vi "airyscan.vi"() -> ()   [LabVIEW 2015]
uses:
  <vilib>/vision/Image Controls.llb/IMAQ Image.ctl
  Control cluster 1.ctl
  Control digital.ctl
  camera.ctl
  <vilib>/vision/NI_Vision_Development_Module.lvlib
panel:
  out "error in (no error) 3":errorcluster
  out "Frame Index":i32
  in  "piezol":T1
  out "output cluster":T2
  in  "stop":bool
  out "picture frame count":i32
  out "one frame#":dbl
  out "image array":T3[](array[typedef])
  out "Image 4":T3(plugin-control)
  out "Slide":u8(slide) scale=0.0..21.0
  out "y width":dbl
  out "x width":dbl
  out "flyback flag":bool=TRUE
  out "actual number of samples written per channel":u32
  out "flyback step":dbl
  out "actual exposure time":dbl
  out "selected path":path
  out "frame #":u16
  out "y#":dbl
  out "x#":dbl
  out "buffer page size":i32
  in  "save":bool
  out "Signal":u32[](array[numeric])
  in  "digital galvo":T4={" galvo offset"=32427.26, "flyback step"=20.0} {"flyback step" min=0.0 max=10.0 step=0.1; "galvo offset" min=0.0 max=10.0 step=0.1}
  in  "p Cluster":T5={"exposure time"=3.8e-05, "frame #"=2, "x#"=512.0, "y#"=512.0, "x step size"=0.0, "y step size"=0.0, "buffer page size"=1000.0} {"buffer page size" min=0.0 max=2044.0 step=4.0; "y step size" format="%.6f"; "x step size" format="%.6f"; "frame #" min=1 max=2048 step=1; "exposure time" min=0.0 max=10.0 step=0.1}
  out "camera handle":u32
  out "buffer array":T3[](array[typedef])
  in  "error in (no error) 2":errorcluster {"code" format="%.0x"}
  out "Camera Details":T6
  in  "abort":bool
  in  "start":bool
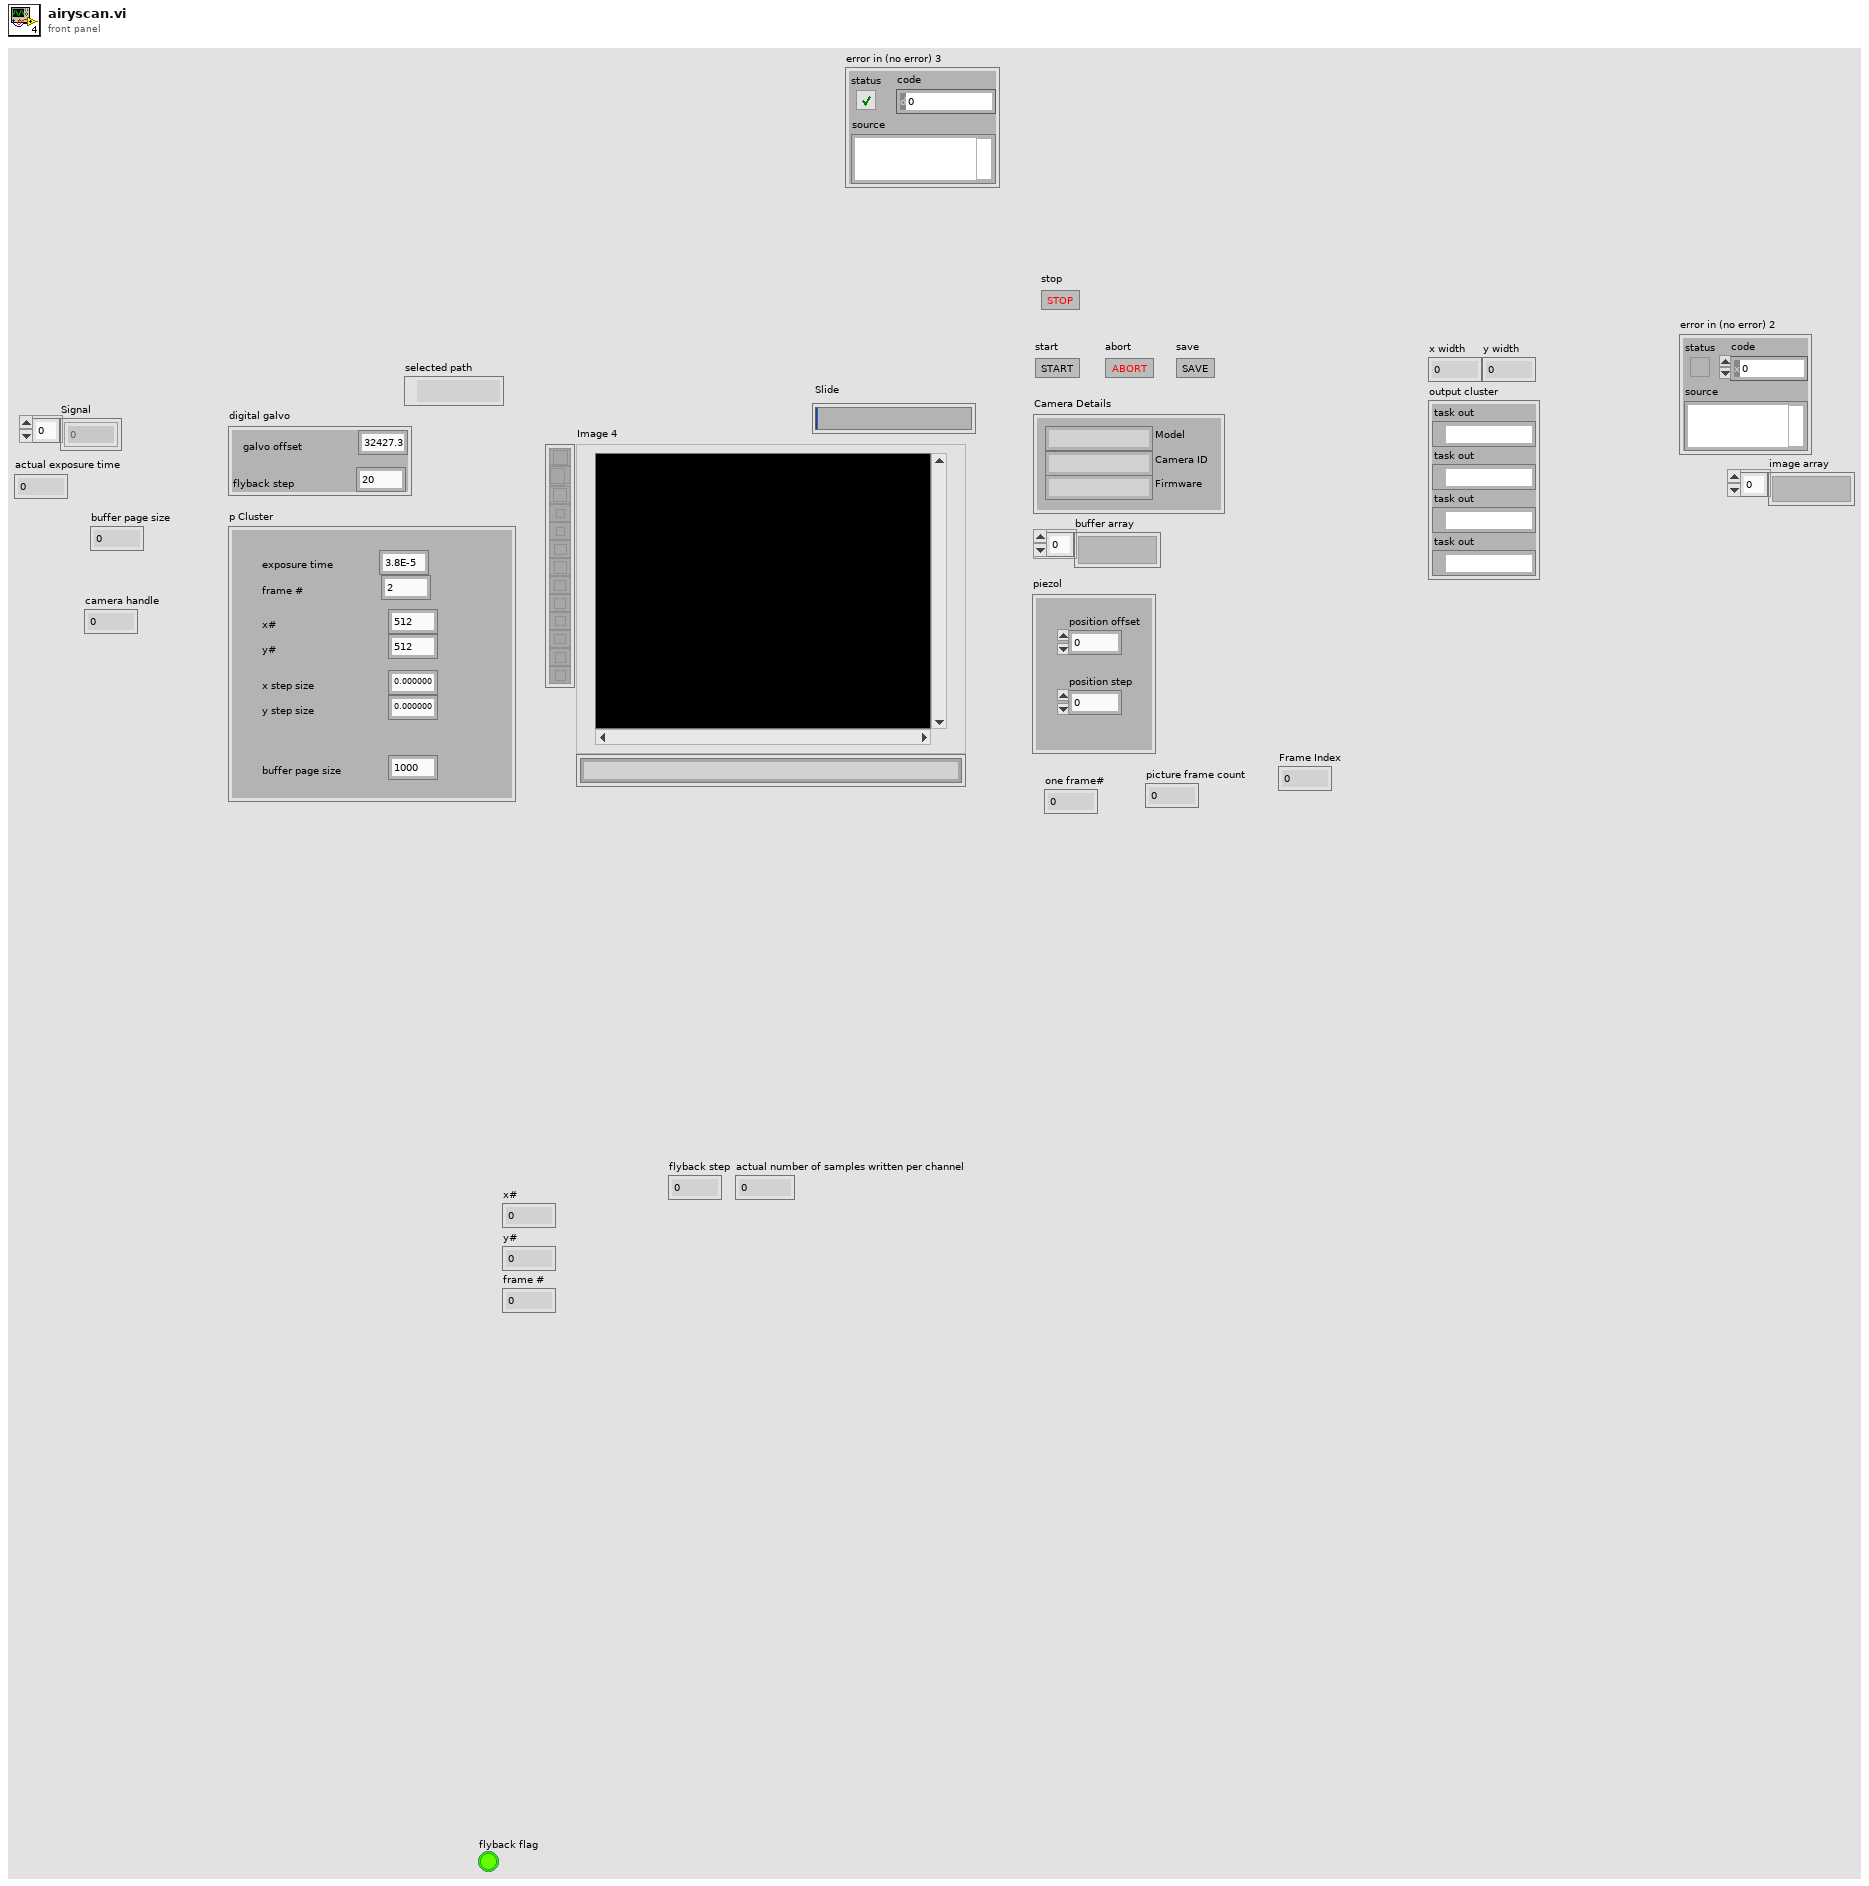
[diagram p1: front panel]
types:
  T1 = cluster{"position offset":dbl, "position step":dbl}
  T2 = cluster{"task out":refnum<k21>, "task out":refnum<k21>, "task out":refnum<k21>, "task out":refnum<k21>}
  T3 = typedef "IMAQ Image.ctl" = refnum<image>
  T4 = typedef "Control digital.ctl" = cluster{" galvo offset":dbl, "flyback step":dbl}
  T5 = typedef "Control cluster 1.ctl" = cluster{"exposure time":dbl, "frame #":u16, "x#":dbl, "y#":dbl, "x step size":dbl, "y step size":dbl, "buffer page size":dbl}
  T6 = cluster{"Model":string, "Camera ID":string, "Firmware":string}
  T7 = typedef "camera.ctl" = enum16{"stop", "state0-initialize", "calculate waveform", "wait for action", "state1-set", "state2-capture", "exit"}
  T8 = cluster{"Rows Per Strip":i32, "Photometric":i32, "Compression Type":i32}
  T9 = typedef "Image Type" = u32
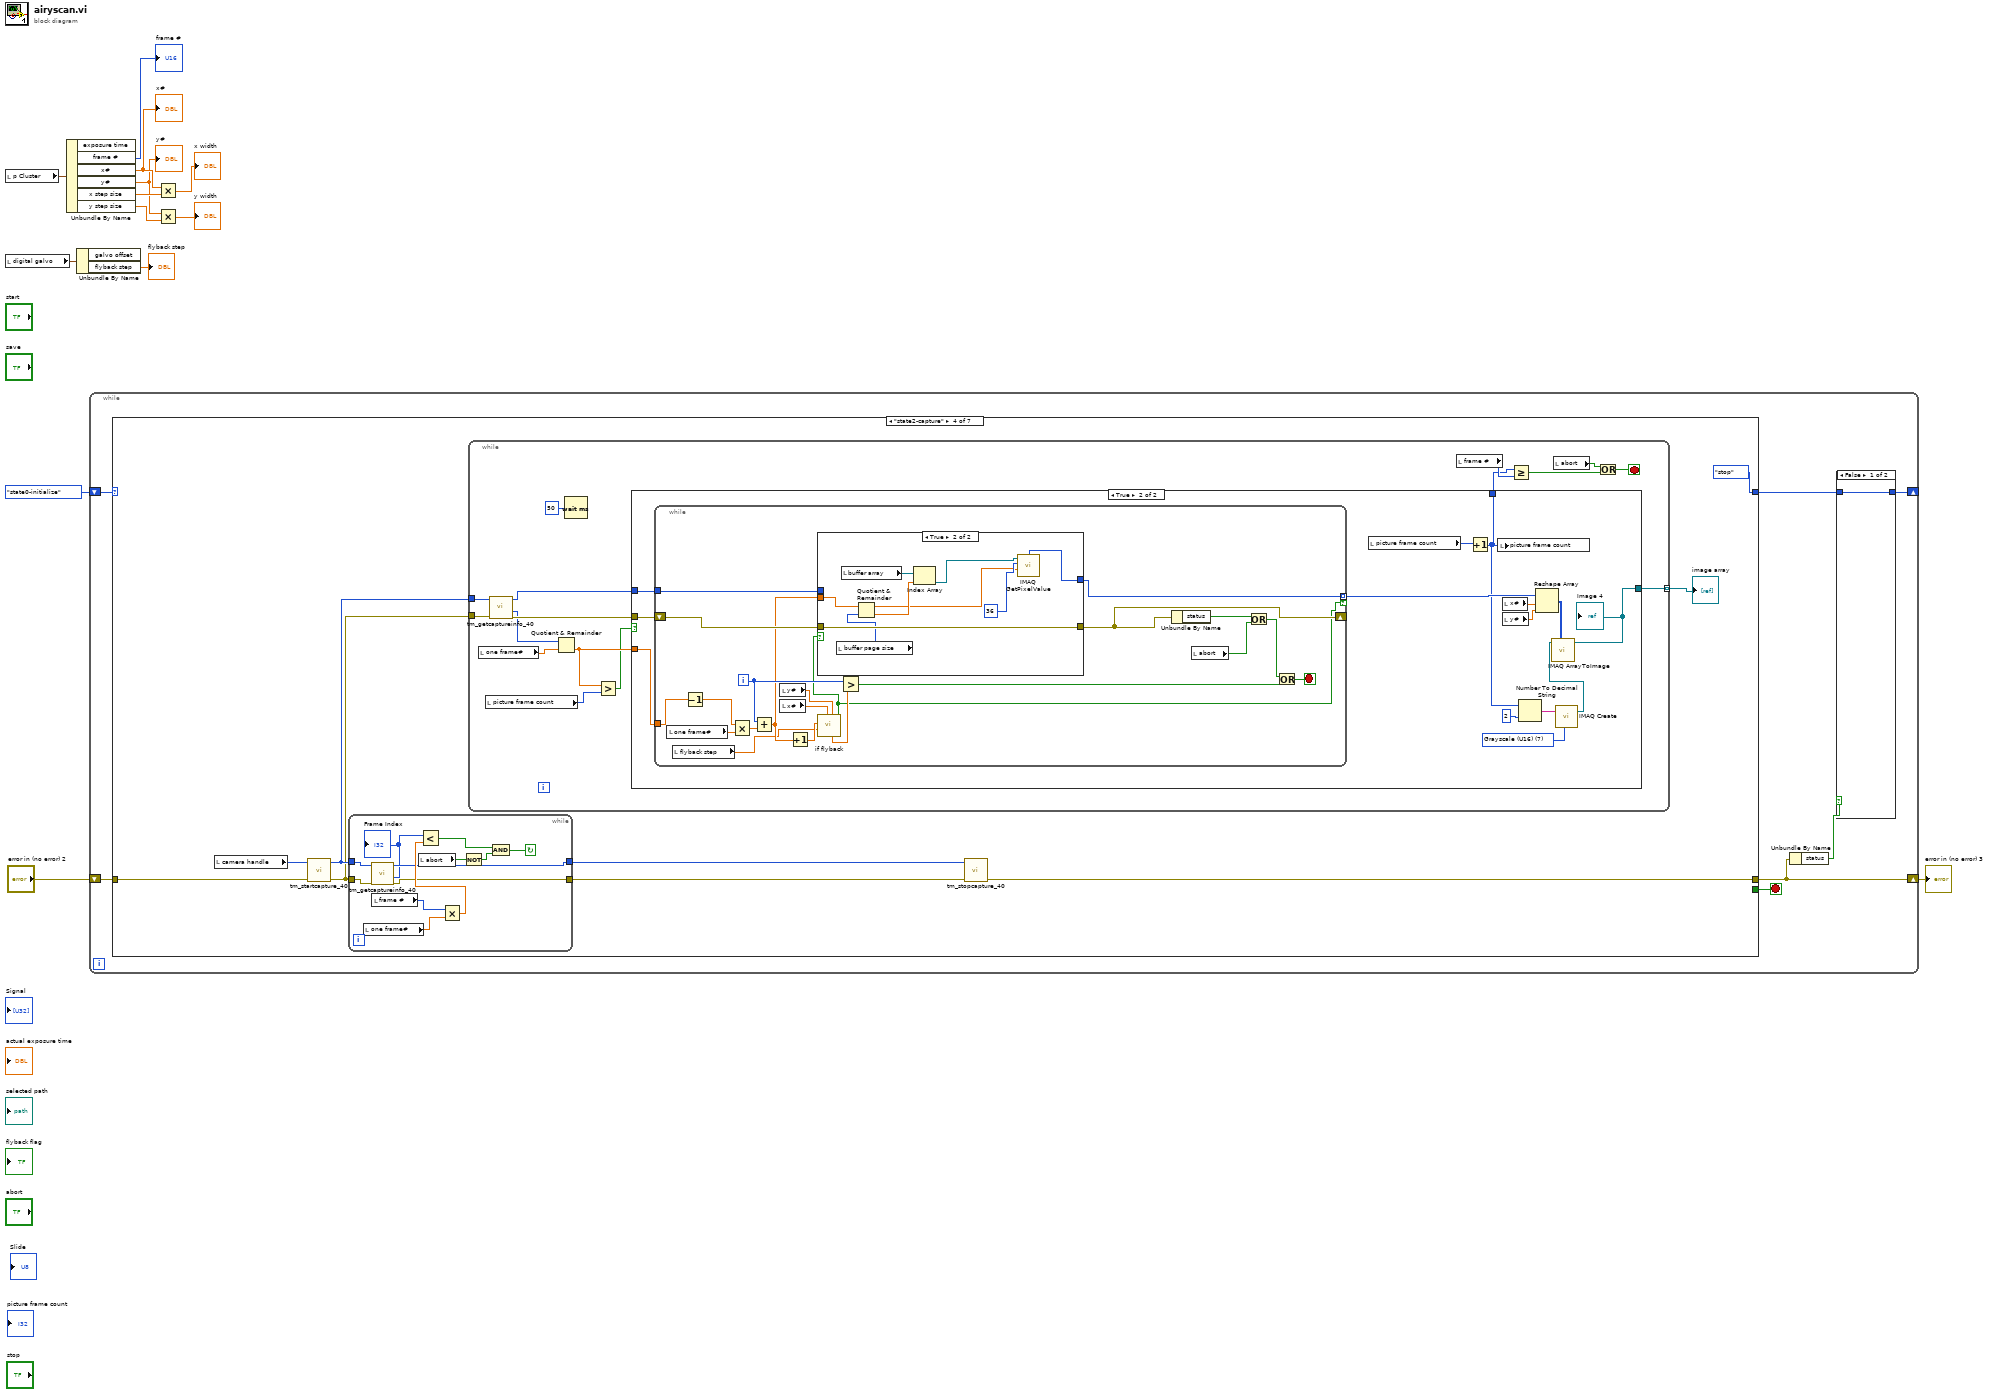
[diagram p0: block diagram]
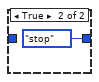
[diagram p2: hidden frame]
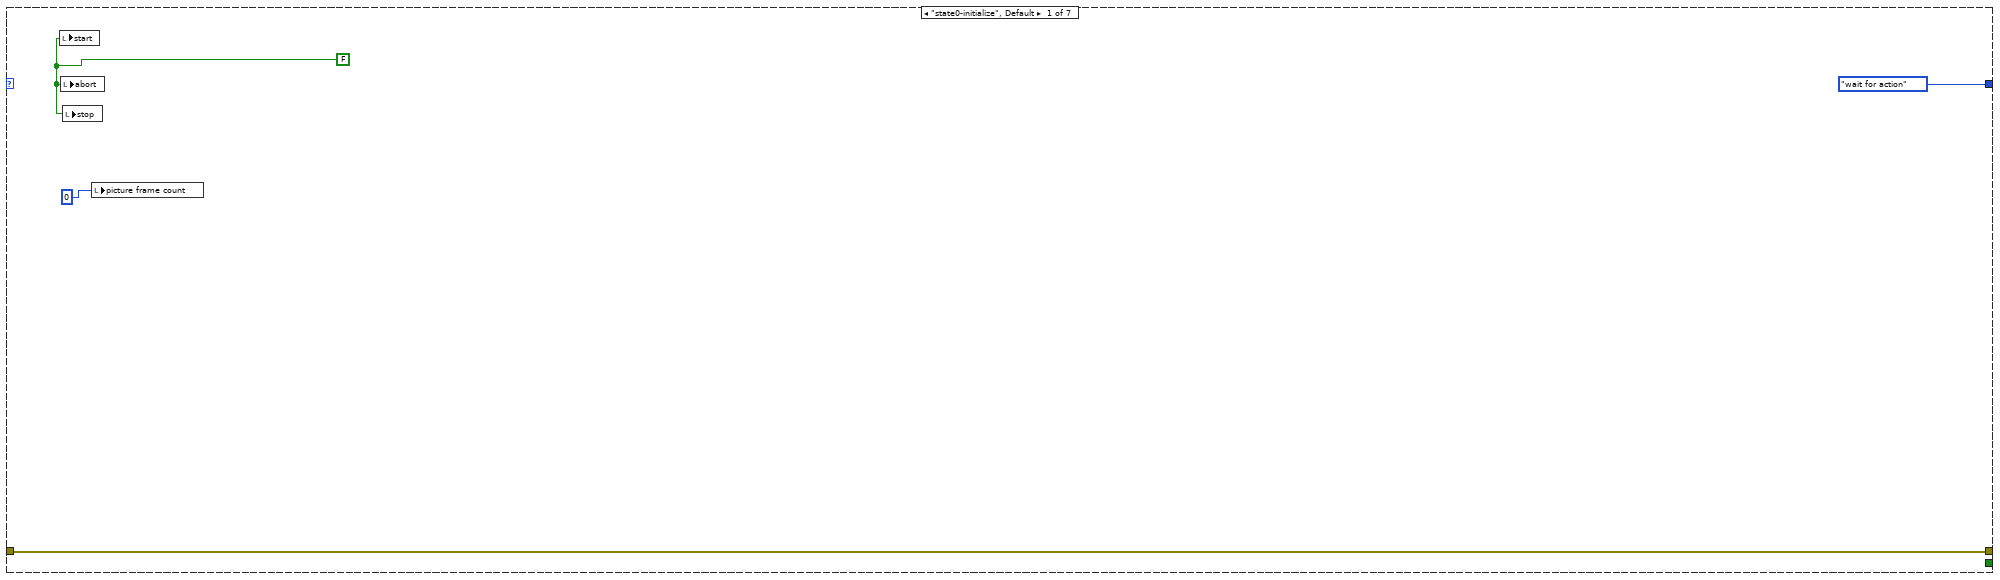
[diagram p3: hidden frame]
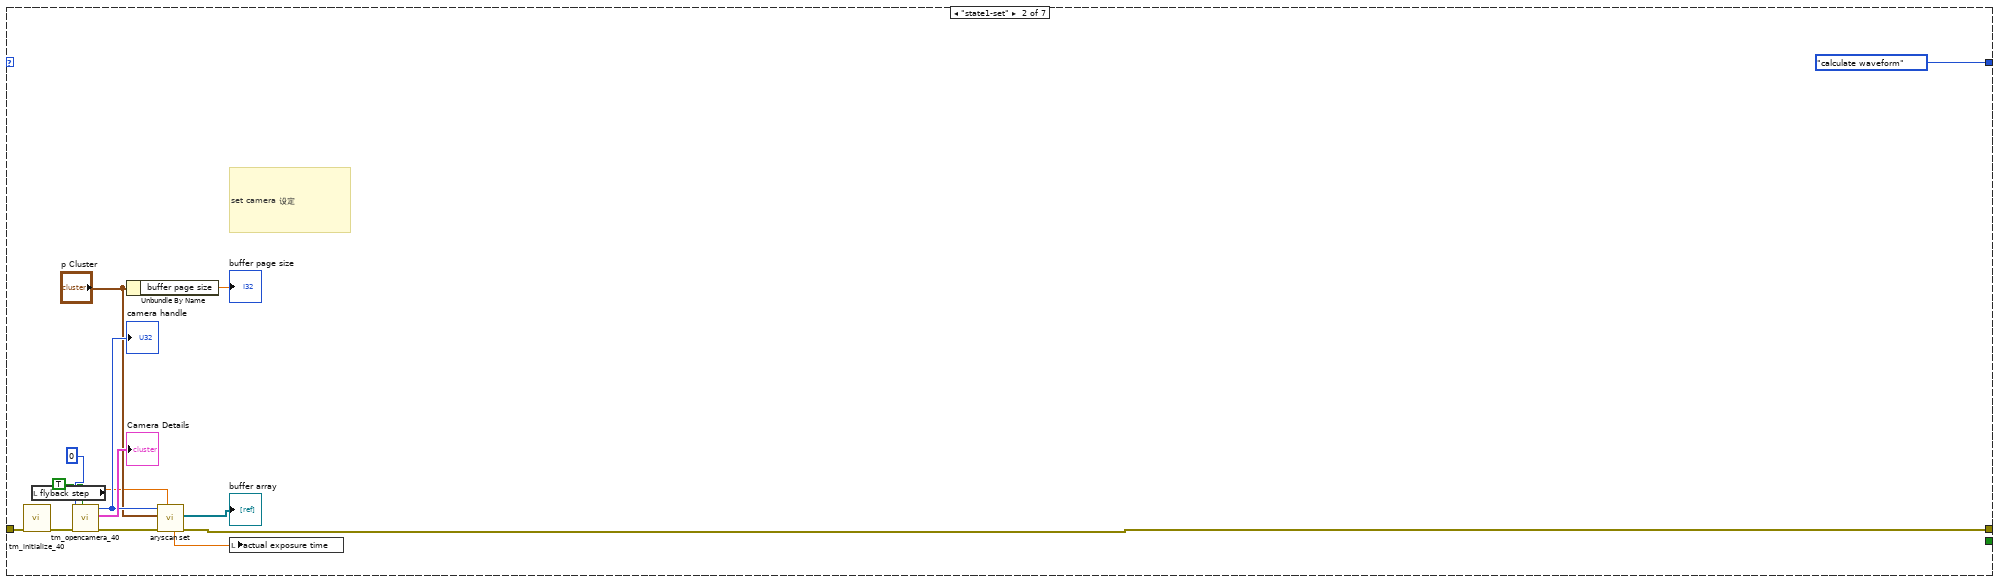
[diagram p4: hidden frame]
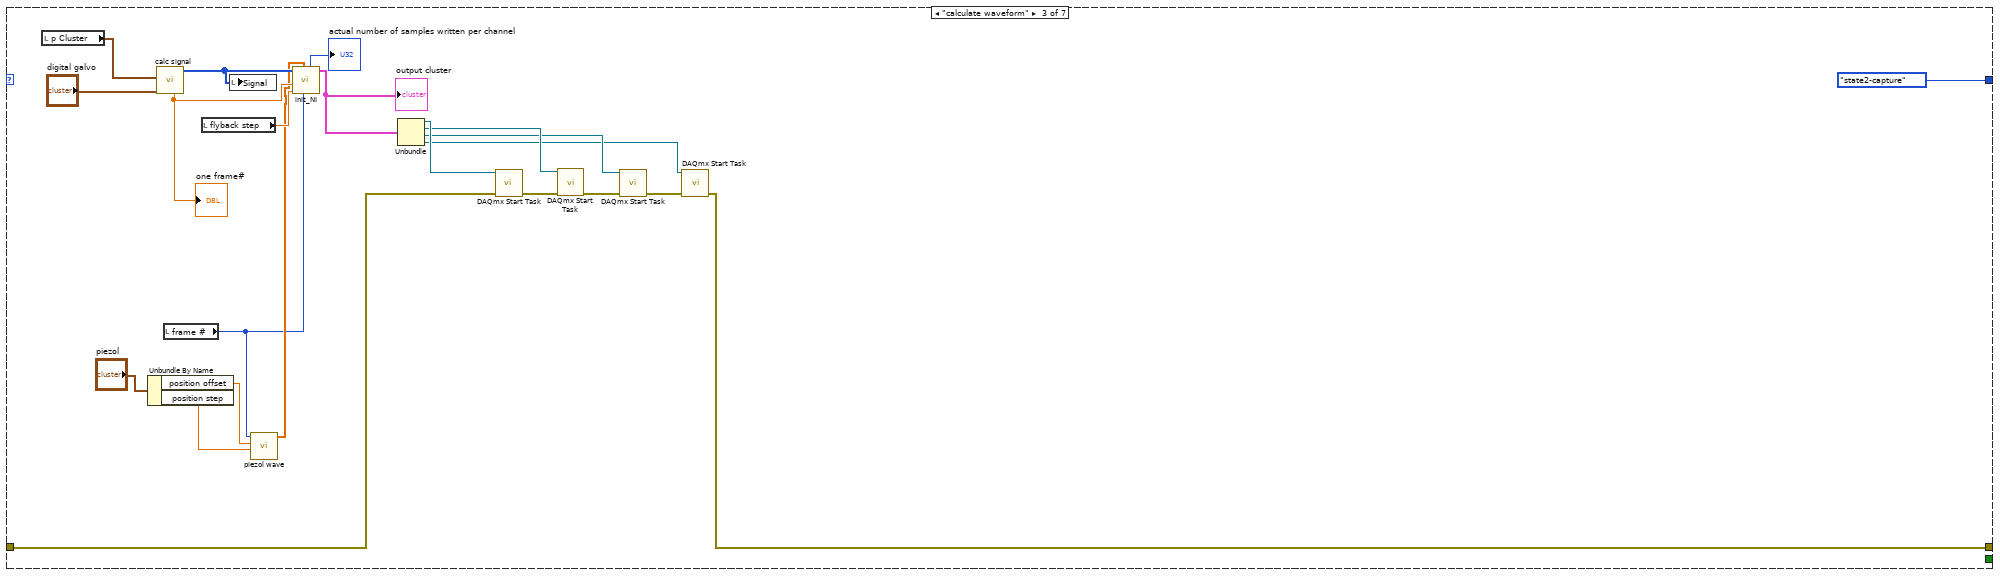
[diagram p5: hidden frame]
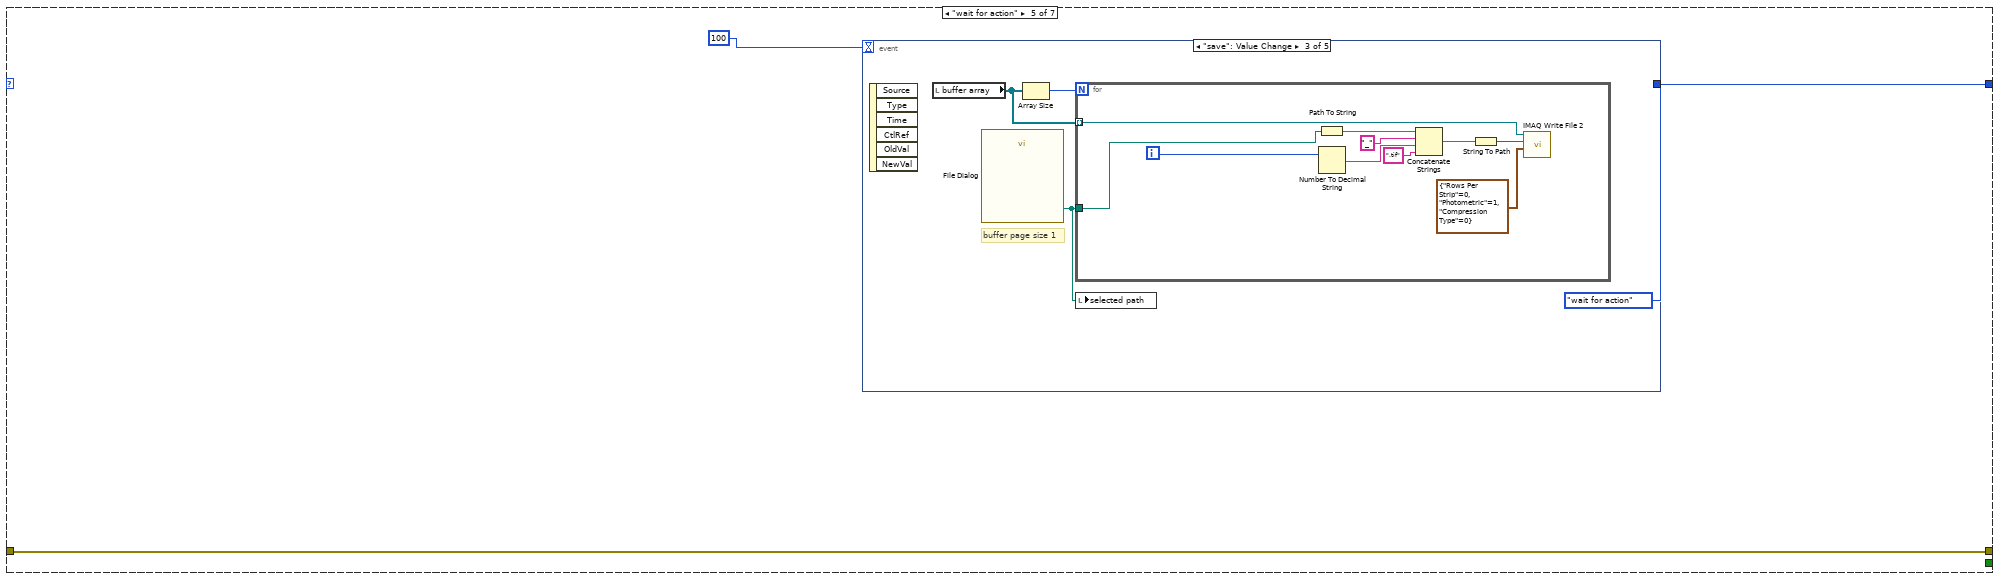
[diagram p8: hidden frame]
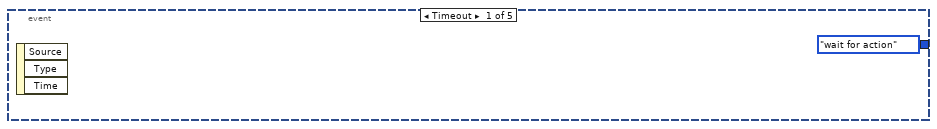
[diagram p9: hidden frame]
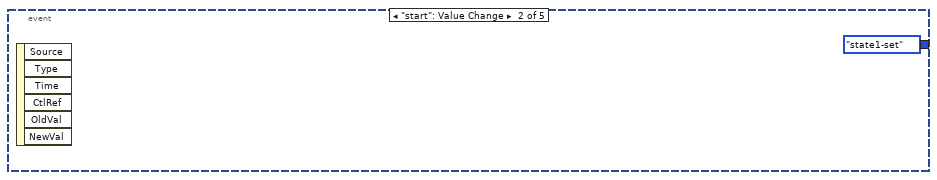
[diagram p10: hidden frame]
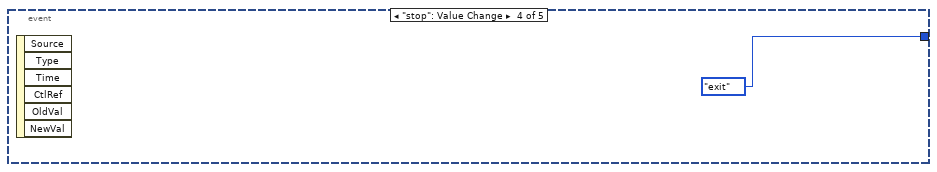
[diagram p11: hidden frame]
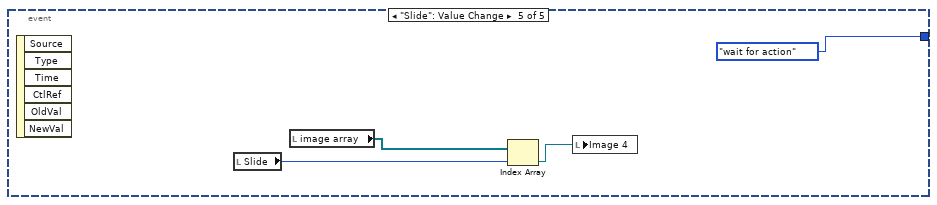
[diagram p12: hidden frame]
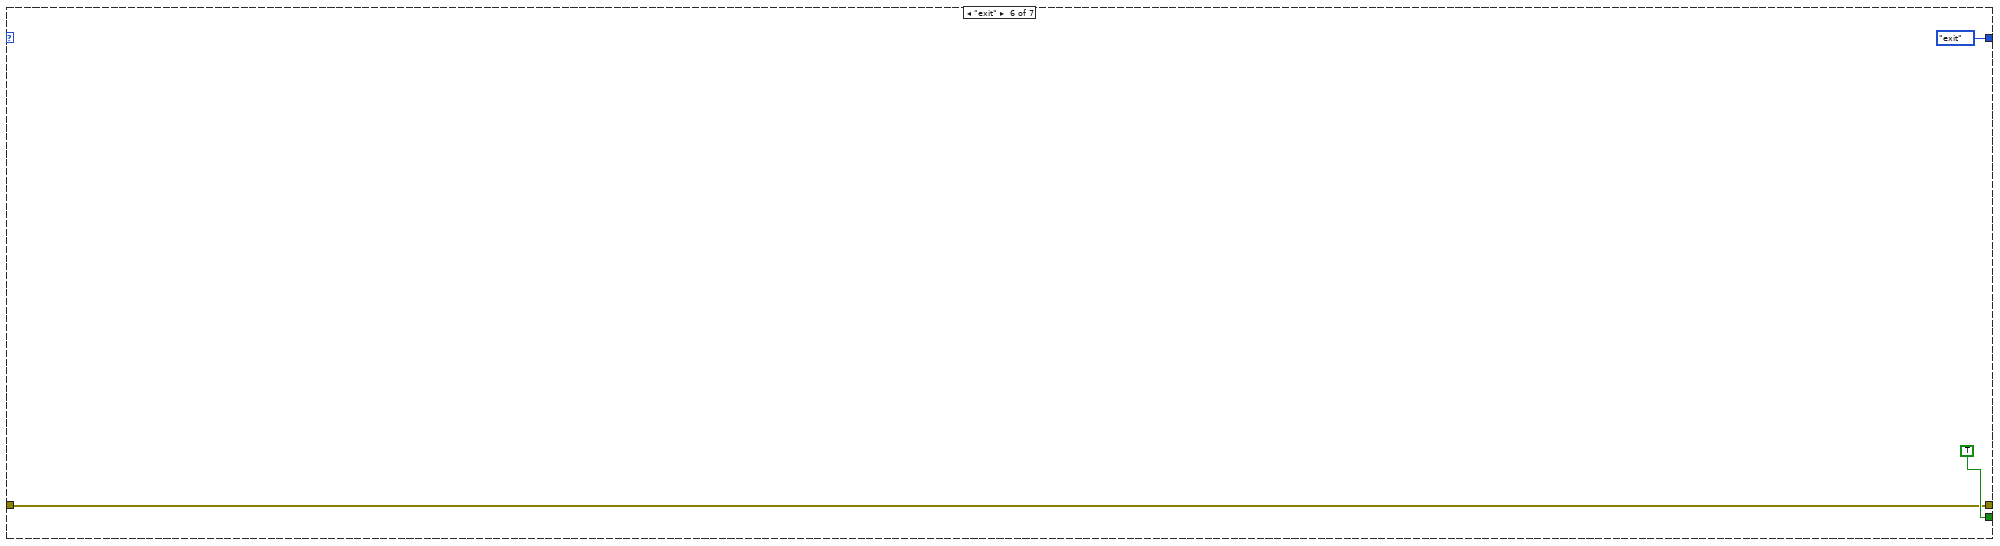
[diagram p13: hidden frame]
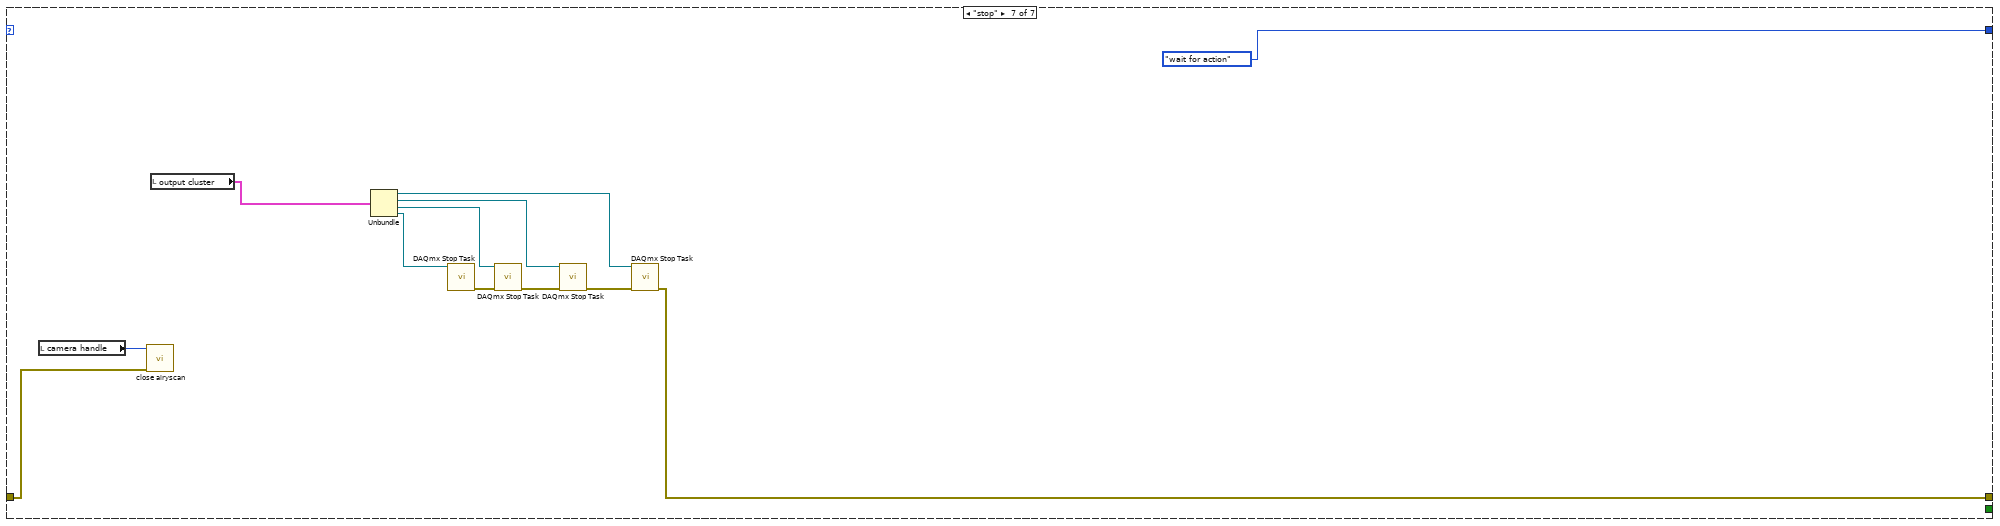
[diagram p14: hidden frame]
diagram:
  n1 = local read "p Cluster"() -> (w10:T5)
  n2 = local read "digital galvo"() -> (w11:T4)
  n3 = Unbundle By Name(w10) -> ("frame #"=→"frame #":u16, "x#"=w3:dbl, "y#"=w2:dbl, "x step size"=w7:dbl, "y step size"=w5:dbl)  [unwired: 1 out]
  "x#" <- w3
  "y#" <- w2
  n4 = Unbundle By Name(w11) -> ("flyback step"=→"flyback step":dbl)  [unwired: 1 out]
  n5 = while {
    shift-right: [w17] -> _
    shift-left: camera."state0-initialize" ("Enum") -> [w14]
    shift-right: [w19] -> w1
    shift-left: "error in (no error) 2" -> [w20]
    stop <- w15 stop-if-true
    n6 = case shown="\"state2-capture\"" w14 {
      tunnel: [camera."wait for action" ("Enum") camera."calculate waveform" ("Enum") camera."state2-capture" ("Enum") camera."stop" ("Enum") w145 camera."exit" ("Enum") camera."wait for action" ("Enum")] -> w16
      tunnel: w20 -> [w26 w38 w47 w70 w147 w169 w174]
      tunnel: [w26 w34 w46 w67 w147 w169 w173] -> w19
      tunnel: [_ _ _ _ _ TRUE _] -> w15
      frame "state0-initialize", Default {
        w23 = FALSE
        n7 = local write "start"(w23) -> ()
        n8 = local write "abort"(w23) -> ()
        n9 = local write "stop"(w23) -> ()
        n10 = local write "picture frame count"(0) -> ()
      }
      frame "state1-set" {
        # "set camera 设定"
        n11 = call <userlib>:"tm_initialize_40.vi"("error in (no error)"=w38) -> ("error out"=w40:errorcluster)  [unwired: 7 in, 3 out]
        n12 = local read "flyback step"() -> (w29:dbl)
        n13 = call <userlib>:"tm_opencamera_40.vi"("Force Open"=TRUE, "error in (no error)"=w40, "Camera Index"=0) -> ("error out"=w35:errorcluster, "Camera Details"=→"Camera Details":T6, "Handle out"=w36:u32)  [unwired: 6 in]
        "camera handle" <- w36
        n14 = Unbundle By Name("p Cluster") -> ("buffer page size"=→"buffer page size":dbl)
        n15 = call "aryscan set.vi"("fly back step #"=w29, "error in (no error)"=w35, "p Cluster"="p Cluster", "Camera handle in"=w36) -> ("error out"=w34:errorcluster, "buffer array"=→"buffer array":T3[], "actual exposure time"=w30:dbl)  [unwired: 4 in, 1 out]
        n16 = local write "actual exposure time"(w30) -> ()
      }
      frame "calculate waveform" {
        n17 = local read "p Cluster"() -> (w61:T5)
        n18 = Unbundle By Name("piezol") -> ("position offset"=w44:dbl, "position step"=w43:dbl)
        n19 = call "calc signal.vi"("digital galvo"="digital galvo", "p Cluster"=w61) -> ("Signal"=w60:u32[], "one frame#"=w57:dbl)  [unwired: 8 in]
        "one frame#" <- w57
        n20 = local read "frame #"() -> (w41:u16)
        n21 = local read "flyback step"() -> (w56:dbl)
        n22 = local write "Signal"(w60) -> ()
        n23 = call "piezol wave.vi"("position step"=w43, "position offset"=w44, "frame#"=w41) -> ("voltage"=w42:dbl[])  [unwired: 8 in]
        n24 = call "init_NI.vi"("frame#"=w41, "Piezol Signal"=w42, "flyback step#"=w56, "one frame#"=w57, "Galvo Signal"=w60) -> ("output cluster"=w55:T2, "actual number of samples written per channel"=→"actual number of samples written per channel":u32)  [unwired: 5 in]
        "output cluster" <- w55
        n25 = Unbundle(w55) -> ("task out"=w54:refnum<k21>, "task out"=w52:refnum<k21>, "task out"=w51:refnum<k21>, "task out"=w48:refnum<k21>)
        n26 = call <vilib>:"DAQmx Start Task.vi"("task/channels in"=w54, "error in"=w47) -> ("error out"=w53:errorcluster)  [unwired: 12 in, 1 out]
        n27 = call <vilib>:"DAQmx Start Task.vi"("task/channels in"=w52, "error in"=w53) -> ("error out"=w50:errorcluster)  [unwired: 12 in, 1 out]
        n28 = call <vilib>:"DAQmx Start Task.vi"("task/channels in"=w51, "error in"=w50) -> ("error out"=w49:errorcluster)  [unwired: 12 in, 1 out]
        n29 = call <vilib>:"DAQmx Start Task.vi"("task/channels in"=w48, "error in"=w49) -> ("error out"=w46:errorcluster)  [unwired: 12 in, 1 out]
      }
      frame "state2-capture" {
        n30 = local read "camera handle"() -> (w71:u32)
        n31 = call <userlib>:"tm_startcapture_40.vi"("error in (no error)"=w70, "Handle in"=w71) -> ("error out"=w65:errorcluster, "Handle out"=w66:u32)  [unwired: 8 in]
        n32 = while {
          tunnel: w66 -> [w141]
          tunnel: w65 -> [w140]
          tunnel: [w135] -> w68
          tunnel: [w134] -> w63
          stop <- w142 continue-if-true
          n33 = local read "one frame#"() -> (w139:dbl)
          n34 = call <userlib>:"tm_getcaptureinfo_40.vi"("error in (no error)"=w140, "Handle in"=w141) -> ("error out"=w134:errorcluster, "Frame Count"=w133:i32, "Handle out"=w135:u32)  [unwired: 6 in, 1 out]
          "Frame Index" <- w133
          n35 = local read "frame #"() -> (w138:u16)
          n36 = local read "abort"() -> (w144:bool)
          n37 = Multiply(x=w138, y=w139) -> (x*y=w137:dbl)
          n38 = Less?(x=w133, y=w137) -> (x < y?=w136:bool)
          n39 = Not(x=w144) -> (.not. x?=w143:bool)
          n40 = And(x=w136, y=w143) -> (x .and. y?=w142:bool)
        }
        n41 = while {
          tunnel: w66 -> [w87]
          tunnel: w65 -> [w86]
          tunnel: [w80] -> w64 mode=indexing
          stop <- w81 stop-if-true
          n42 = local read "one frame#"() -> (w79:dbl)
          n43 = local read "picture frame count"() -> (w78:i32)
          n44 = call <userlib>:"tm_getcaptureinfo_40.vi"("error in (no error)"=w86, "Handle in"=w87) -> ("error out"=w85:errorcluster, "Frame Count"=w72:i32, "Handle out"=w73:u32)  [unwired: 6 in, 1 out]
          n45 = Quotient & Remainder(x=w72, y=w79) -> (floor(x/y)=w77:dbl)  [unwired: 1 out]
          n46 = Wait (ms)(milliseconds to wait=u32 50) -> ()  [unwired: 1 out]
          n47 = Greater?(x=w77, y=w78) -> (0:w76:bool)
          n48 = case shown="True" w76 {
            tunnel: w85 -> [_ w93]
            tunnel: [_ w92] -> w80
            tunnel: w77 -> [_ w91]
            tunnel: [_ w89] -> w75
            tunnel: w73 -> [_ w88]
            frame False {
            }
            frame True {
              w97 = T9 7 items=["Grayscale (U8)", "Grayscale (I16)", "Grayscale (SGL)", "Complex (CSG)", "RGB (U32)", "HSL (U32)", "RGB (U64)", "Grayscale (U16)"] ("Image Type")
              n49 = while {
                shift-right: [w117] -> _
                shift-left: w93 -> [w118]
                tunnel: [w107] -> w96 mode=indexing if=w106
                tunnel: w91 -> [w109]
                tunnel: w88 -> [w105]
                i -> [w110]
                stop <- w116 stop-if-true
                n50 = local read "one frame#"() -> (w112:dbl)
                n51 = local read "flyback step"() -> (w102:dbl)
                n52 = Decrement(x=w109) -> (x-1=w108:dbl)
                n53 = Multiply(x=w108, y=w112) -> (x*y=w111:dbl)
                n54 = Add(x=w110, y=w111) -> (x+y=w104:dbl)
                n55 = local read "y#"() -> (w121:dbl)
                n56 = local read "x#"() -> (w120:dbl)
                n57 = Increment(x=w104) -> (x+1=w103:dbl)
                n58 = call "if flyback.vi"("y#"=w121, "x#"=w120, "flyback step#"=w102, "frame count"=w103) -> ("save?"=w106:bool, "one frame #"=w114:dbl)  [unwired: 6 in]
                n59 = case shown="True" w106 {
                  tunnel: w104 -> [_ w131]
                  tunnel: w118 -> [w123 w132]
                  tunnel: [w123 w132] -> w117
                  tunnel: [_ w130] -> w107
                  tunnel: w105 -> [_ _]
                  frame False {
                  }
                  frame True {
                    n60 = local read "buffer page size"() -> (w128:i32)
                    n61 = local read "buffer array"() -> (w129:T3[])
                    n62 = Quotient & Remainder(x=w131, y=w128) -> (x-y*floor(x/y)=w124:dbl, floor(x/y)=w127:dbl)
                    n63 = Index Array(array=w129, index=w127) -> (element=w126:T3)
                    n64 = call "IMAQ GetPixelValue"("Image"=w126, "X Coordinate"=36, "Y Coordinate"=w124) -> ("Pixel Value (U16)"=w130:u16)  [unwired: 3 in, 4 out]
                  }
                }
                n65 = Greater?(x=w110, y=w114) -> (0:w113:bool)
                n66 = Unbundle By Name(w117) -> ("status"=w122:bool)
                n67 = local read "abort"() -> (w115:bool)
                n68 = Or(x=w122, y=w115) -> (x .or. y?=w119:bool)
                n69 = Or(x=w119, y=w113) -> (x .or. y?=w116:bool)
              }
              n70 = local read "picture frame count"() -> (w90:i32)
              n71 = Increment(x=w90) -> (x+1=w89:i32)
              n72 = local write "picture frame count"(w89) -> ()
              n73 = local read "x#"() -> (w95:dbl)
              n74 = local read "y#"() -> (w94:dbl)
              n75 = Number To Decimal String(number=w89, width (-)=i16 2) -> (decimal integer string=w100:string)
              n76 = Reshape Array(w96, w95, w94) -> (w98:u16[][])
              n77 = call "IMAQ Create"("Image Name"=w100, "Image Type"=w97) -> ("New Image"=w99:T3)  [unwired: 3 in, 1 out]
              n78 = call "IMAQ ArrayToImage"("Image Pixels (U16)"=w98, "Image"=w99) -> ("Image Out"=w92:T3)  [unwired: 8 in, 1 out]
              "Image 4" <- w92
            }
          }
          n79 = local read "frame #"() -> (w84:u16)
          n80 = Greater Or Equal?(x=w75, y=w84) -> (x >= y?=w83:bool)
          n81 = local read "abort"() -> (w82:bool)
          n82 = Or(x=w82, y=w83) -> (x .or. y?=w81:bool)
        }
        "image array" <- w64
        n83 = call <userlib>:"tm_stopcapture_40.vi"("error in (no error)"=w63, "Handle in"=w68) -> ("error out"=w67:errorcluster)  [unwired: 8 in, 1 out]
      }
      frame "wait for action" {
        n84 = event shown="[2] \"save\": Value Change" {
          selector: _ -> [_ _ _ _ _]
          dyn-events: _ -> [_ _ _ _ _]
          timeout: 100 -> [_ _ _ _ _]
          tunnel: [camera."wait for action" ("Enum") camera."state1-set" ("Enum") camera."wait for action" ("Enum") camera."exit" ("Enum") camera."wait for action" ("Enum")] -> w145
          event Timeout {
            n85 = event-data() -> ()  [unwired: 1 in, 3 out]
          }
          event "start": Value Change {
            n86 = event-data() -> ()  [unwired: 1 in, 6 out]
          }
          event "save": Value Change {
            # "buffer page size 1"
            n87 = event-data() -> ()  [unwired: 1 in, 6 out]
            n88 = local read "buffer array"() -> (w152:T3[])
            n89 = call "File Dialog"() -> ("selected path"=w151:path)  [unwired: 12 in, 3 out]
            n90 = Array Size(array=w152) -> (size(s)=w150:i32)
            n91 = for {
              N: w150 -> [_]
              tunnel: w152 -> [w162] mode=indexing
              tunnel: w151 -> [w163]
              i -> [w161]
              n92 = Path To String(path=w163) -> (string=w158:string)
              n93 = Number To Decimal String(number=w161) -> (decimal integer string=w159:string)  [unwired: 1 in]
              n94 = Concatenate Strings(w158, "_", w159, ".tif" ("string")) -> (w155:string)
              n95 = String To Path(string=w155) -> (path=w156:path)
              n96 = call-poly "IMAQ Write File 2"("TIFF Options"=T8 {"Rows Per Strip"=0, "Photometric"=1, "Compression Type"=0}, "File Path"=w156, "Image"=w162) -> ()  [unwired: 7 in, 2 out]
            }
            n97 = local write "selected path"(w151) -> ()
          }
          event "stop": Value Change {
            n98 = event-data() -> ()  [unwired: 1 in, 6 out]
          }
          event "Slide": Value Change {
            n99 = event-data() -> ()  [unwired: 1 in, 6 out]
            n100 = local read "Slide"() -> (w168:u8)
            n101 = local read "image array"() -> (w167:T3[])
            n102 = Index Array(array=w167, index=w168) -> (element=w166:T3)
            n103 = local write "Image 4"(w166) -> ()
          }
        }
      }
      frame "exit" {
      }
      frame "stop" {
        n104 = local read "camera handle"() -> (w183:u32)
        n105 = call "close airyscan.vi"("error in (no error)"=w174, "camera handle"=w183) -> ()  [unwired: 9 in, 1 out]
        n106 = local read "output cluster"() -> (w182:T2)
        n107 = Unbundle(w182) -> ("task out"=w178:refnum<k21>, "task out"=w179:refnum<k21>, "task out"=w180:refnum<k21>, "task out"=w181:refnum<k21>)
        n108 = call <vilib>:"DAQmx Stop Task.vi"("task/channels in"=w181) -> ("error out"=w177:errorcluster)  [unwired: 13 in, 1 out]
        n109 = call <vilib>:"DAQmx Stop Task.vi"("task/channels in"=w180, "error in"=w177) -> ("error out"=w176:errorcluster)  [unwired: 12 in, 1 out]
        n110 = call <vilib>:"DAQmx Stop Task.vi"("task/channels in"=w179, "error in"=w176) -> ("error out"=w175:errorcluster)  [unwired: 12 in, 1 out]
        n111 = call <vilib>:"DAQmx Stop Task.vi"("task/channels in"=w178, "error in"=w175) -> ("error out"=w173:errorcluster)  [unwired: 12 in, 1 out]
      }
    }
    n112 = Unbundle By Name(w19) -> ("status"=w18:bool)
    n113 = case shown="False" w18 {
      tunnel: [w21 camera."stop" ("Enum")] -> w17
      tunnel: w16 -> [w21 _]
      frame False {
      }
      frame True {
      }
    }
  }
  "error in (no error) 3" <- w1
  n114 = Multiply(x=w3, y=w7) -> (x*y=→"x width":dbl)
  n115 = Multiply(x=w2, y=w5) -> (x*y=→"y width":dbl)
